vi "GetScans.vi"(6 "condition":string, 7 "error in (no error)":errorcluster, 8 "exp_date":string, 9 "mouse_id":dbl, 10 "Database in":refnum<class "Database.lvclass">) -> (0 "error out":errorcluster, 2 "Scan Clusters":T1(array[cluster]), 3 "Database out":refnum<class "Database.lvclass">, 5 "data":variant[][](array[variant]))   [LabVIEW 2013, in "Database.lvclass"]
uses:
  Database.lvclass
  Database.lvclass/Database.ctl
  <vilib>/addons/database/_DB Variant To Data/Database Variant To Data.xnode
  <vilib>/addons/database/NI_Database_API.lvlib
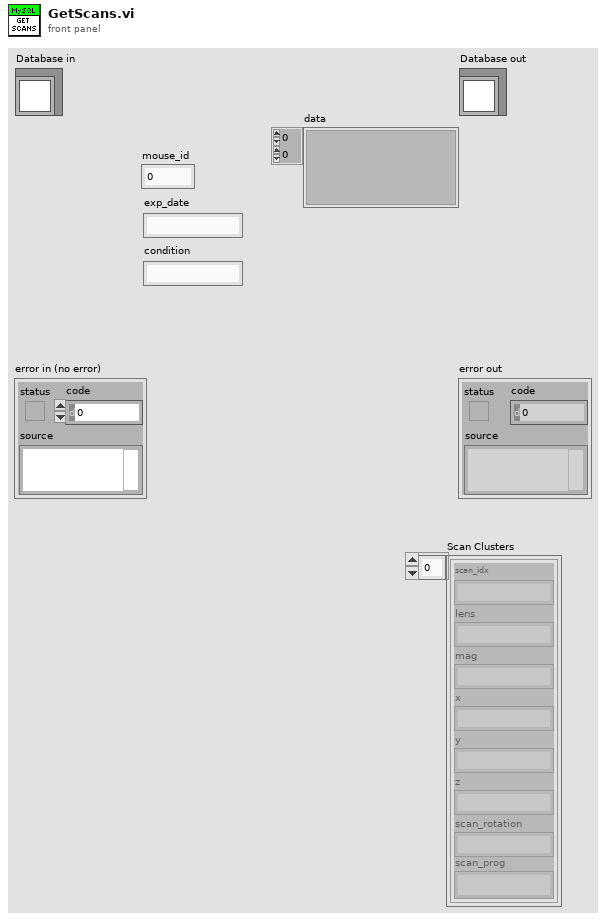
[diagram p1: front panel]
types:
  T1 = cluster{"scan_idx":string, "lens":string, "mag":string, "x":string, "y":string, "z":string, "scan_rotation":string, "scan_prog":string}[]
  T2 = typedef "NI_Database_API.lvlib/Conn ObjectReference.ctl" = refnum<k1>
  T3 = cluster{"data[0]":string, "data[1]":string, "data[2]":string, "data[3]":string, "data[4]":string, "data[5]":string, "data[6]":string, "data[7]":string}
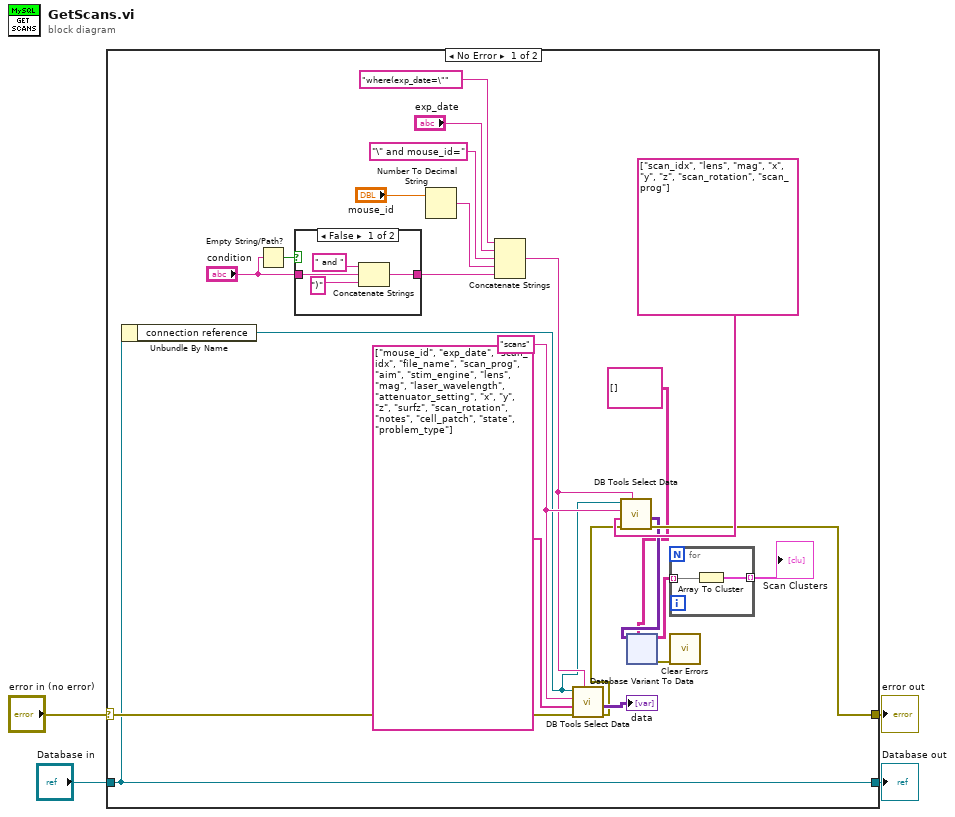
[diagram p0: block diagram]
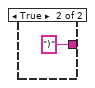
[diagram p2: hidden frame]
diagram:
  n1 = case shown="No Error" "error in (no error)" {
    selector: "error in (no error)" -> [w27 w80]
    tunnel: [w9 w80] -> w3
    tunnel: [w21 w79] -> w1
    tunnel: "Database in" -> [w21 w79]
    frame No Error {
      w13 = "scans" ("table")
      n2 = Unbundle By Name(w21) -> ("connection reference"=w7:T2)
      n3 = Empty String/Path?(string/path="condition") -> (empty?=w17:bool)
      n4 = case shown="False" w17 {
        tunnel: [w28 ")"] -> w18
        tunnel: "condition" -> [w30 _]
        frame False {
          n5 = Concatenate Strings(" and " ("string"), w30, ")" ("string")) -> (w28:string)
        }
        frame True {
        }
      }
      n6 = Number To Decimal String(number="mouse_id") -> (decimal integer string=w23:string)  [unwired: 1 in]
      n7 = Concatenate Strings("where(exp_date=\"", "exp_date", "\" and mouse_id=", w23, w18) -> (w12:string)
      n8 = call <vilib>:"DB Tools Select Data.vi"("condition"=w12, "error in (no error)"=w27, "columns"=string[] ["mouse_id", "exp_date", "scan_idx", "file_name", "scan_prog", "aim", "stim_engine", "lens", "mag", "laser_wavelength", "attenuator_setting", "x", "y", "z", "surfz", "scan_rotation", "notes", "cell_patch", "state", "problem_type"], "table"=w13, "connection reference"=w7) -> ("error out"=w10:errorcluster, "data"=→"data":variant[][])  [unwired: 1 in, 1 out]
      n9 = call <vilib>:"DB Tools Select Data.vi"("condition"=w12, "error in (no error)"=w10, "columns"=string[] ["scan_idx", "lens", "mag", "x", "y", "z", "scan_rotation", "scan_prog"], "table"=w13, "connection reference"=w7) -> ("error out"=w9:errorcluster, "data"=w8:variant[][])  [unwired: 1 in, 1 out]
      n10 = xnode "Database Variant To Data"("database variant"=w8, "type"=string[][] []) -> ("data"=w20:string[][], "error out"=w15:errorcluster)  [unwired: 1 in]
      n11 = for {
        tunnel: w20 -> [w34] mode=indexing
        tunnel: [w33] -> w5 mode=indexing
        n12 = Array To Cluster(array=w34) -> (cluster=w33:T3)
      }
      "Scan Clusters" <- w5
      n13 = call <vilib>:"Clear Errors.vi"("error in (no error)"=w15) -> ()  [unwired: 6 in, 1 out]
    }
    frame Error {
    }
  }
  "error out" <- w3
  "Database out" <- w1
